vi "SDK Test x64.vi"() -> ()   [LabVIEW 2014]
panel:
  in  "Select Filter Wheel":i32(ring)=1 items=["Filter Wheel 1", "Filter Wheel 2"]
  in  "Select mirror":i32(ring)=1 items=["Mirror 1", "Mirror 2"]
  out "Pixel calibration":dbl
  out "XY Graph":cluster{"Y":dbl[], "Y":dbl[]}[](graph)
  in  "Get calibration":bool
  in  "Pixel Index":i32
  in  "Pixel Width":dbl
  in  "Central WL":dbl
  in  "Pixel Count":i32
  in  "Central Pixel":i32
  out "?":i32
  in  "Grating count":bool
  out "Grating":i32
  in  "Get active grating":bool
  in  "Set active grating":bool
  out "Max WL":dbl
  out "Min WL":dbl
  out "Grooves":i32
  in  "Grating":i32(ring) items=["Grating 1", "Grating 2", "Grating 3", "Grating 4"]
  in  "Reset active grating":bool
  out "Dispersion":dbl format="%.4f"
  out "Error":string
  out "Cur. state":i32(ring) items=["Unknown", "Open", "Close"]
  in  "Set shutter state":bool
  in  "Select shutter state":u32(ring) items=["Open", "Close"]
  out "Cur. filter":i32(ring) items=["Filter1", "Filter2", "Filter3", "Filter4", "Filter5", "Filter6", "Filter7", "Filter8"]
  in  "Set filter":bool
  in  "Select filter state":i32(ring) items=["Filter1", "Filter2", "Filter3", "Filter4", "Filter5", "Filter6", "Filter7", "Filter8"]
  out "Cur. mirror":i32(ring) items=["Undefined"=-1, "Axial port"=0, "Lateral port"=1]
  in  "Set mirror":bool
  in  "Select mirror state":i32(ring)=1 items=["Axial port"=1, "Lateral port"=2]
  in  "Reset":bool
  in  "Set slit width":bool
  out "Slit width":dbl format="%.2f"
  in  "Select slit":i32(ring) items=["Slit 1", "Slit 2", "Slit 3", "Slit 4"]
  in  "New slit width":dbl format="%.2f"
  in  "Stop control":bool
  in  "Set new WL":bool caption="Boolean"
  out "Cur WL":dbl format="%.2f"
  in  "New WL":dbl format="%.2f"
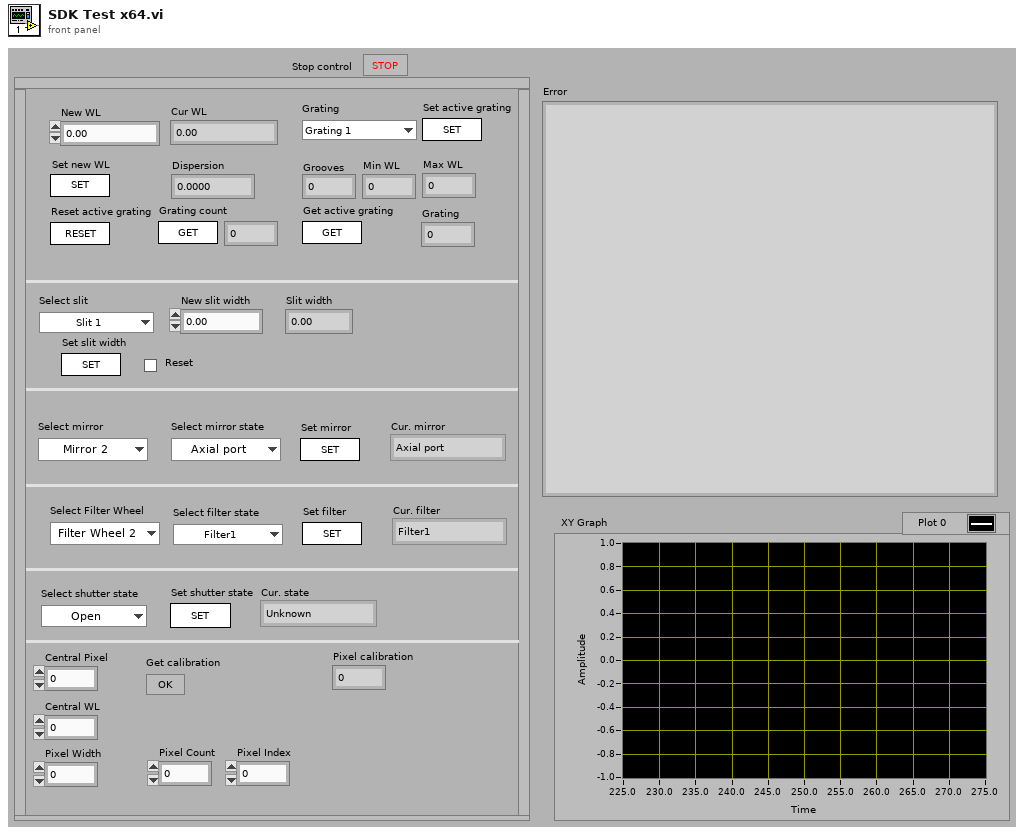
[diagram p1: front panel]
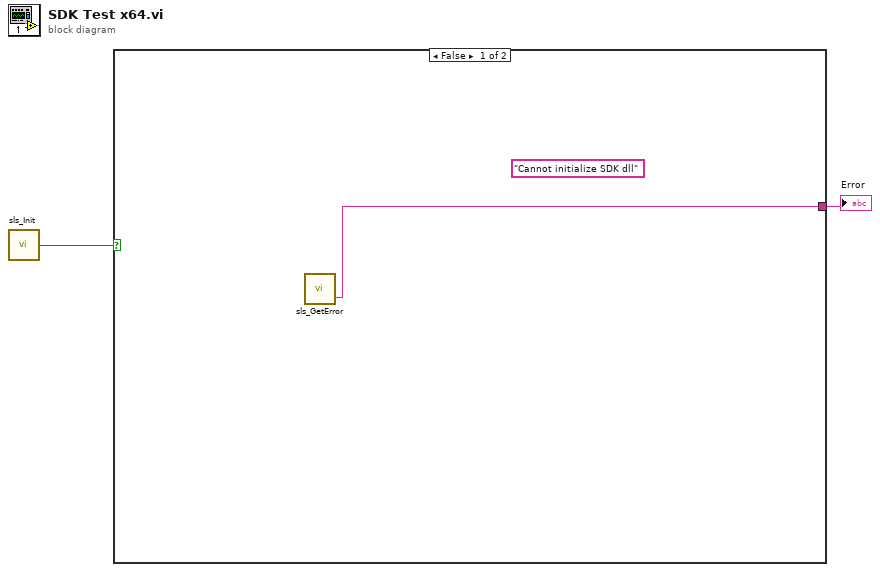
[diagram p0: block diagram]
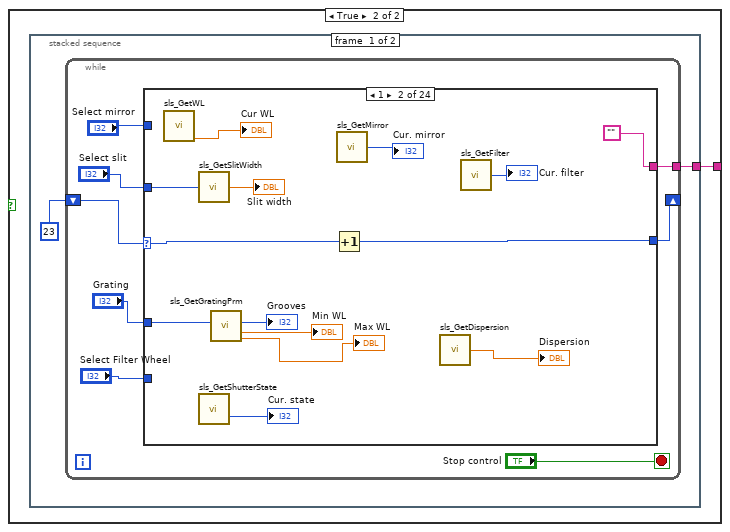
[diagram p2: hidden frame]
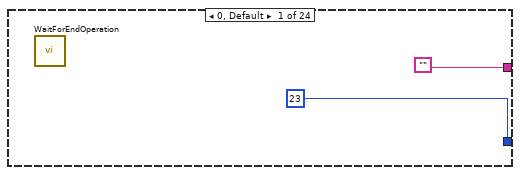
[diagram p3: hidden frame]
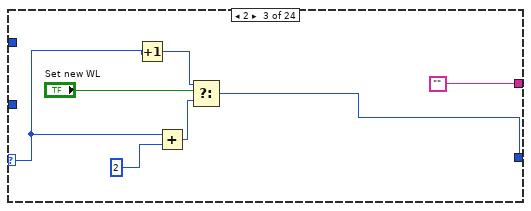
[diagram p4: hidden frame]
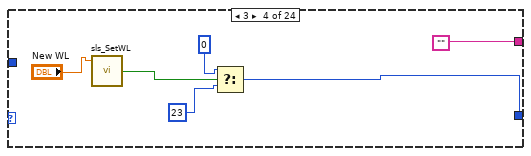
[diagram p5: hidden frame]
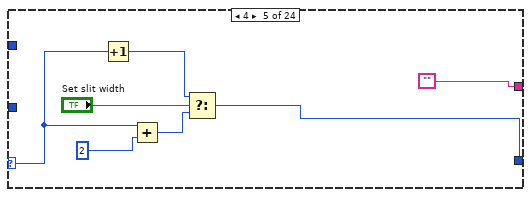
[diagram p6: hidden frame]
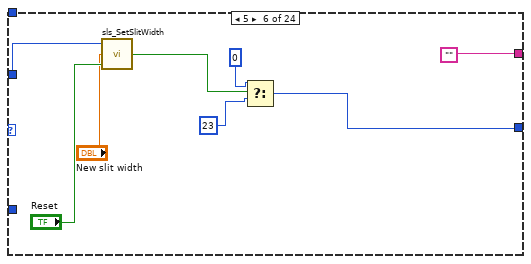
[diagram p7: hidden frame]
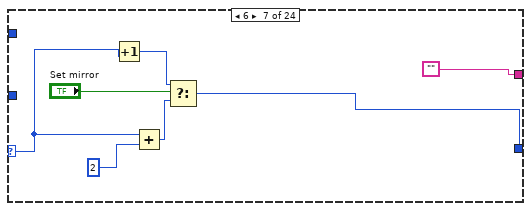
[diagram p8: hidden frame]
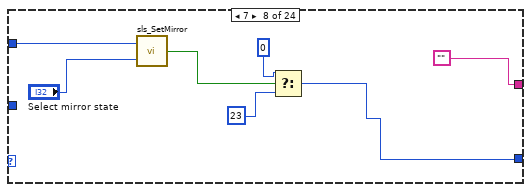
[diagram p9: hidden frame]
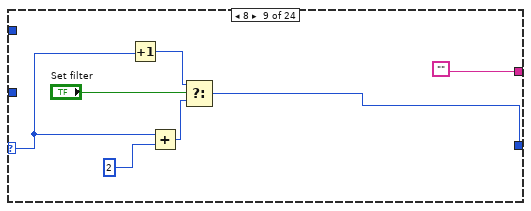
[diagram p10: hidden frame]
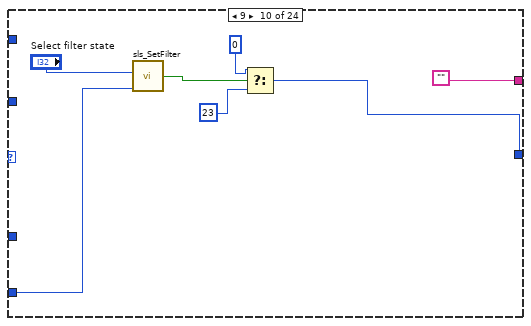
[diagram p11: hidden frame]
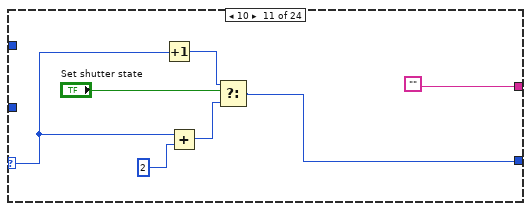
[diagram p12: hidden frame]
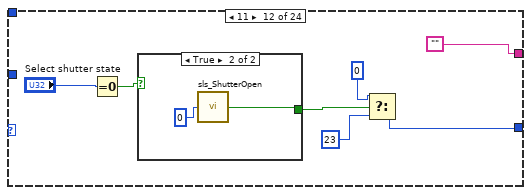
[diagram p13: hidden frame]
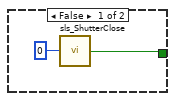
[diagram p14: hidden frame]
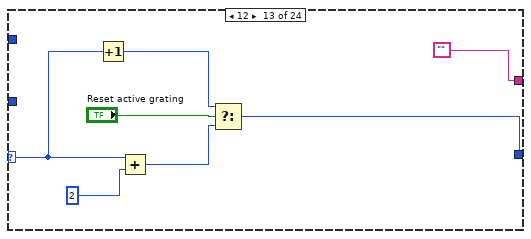
[diagram p15: hidden frame]
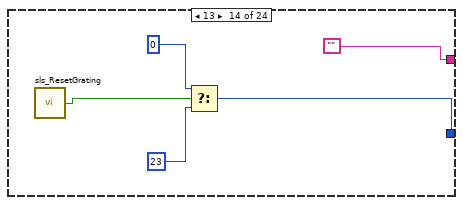
[diagram p16: hidden frame]
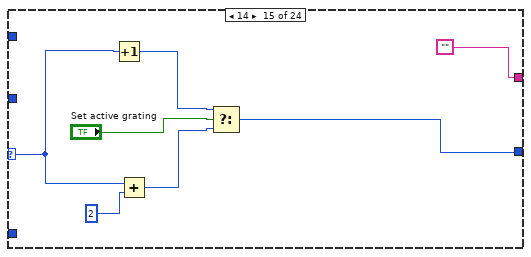
[diagram p17: hidden frame]
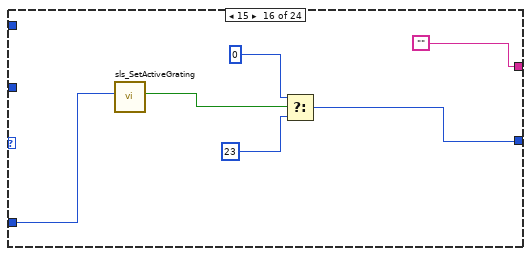
[diagram p18: hidden frame]
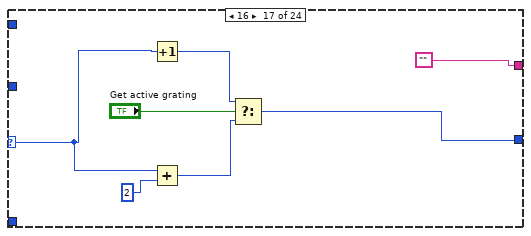
[diagram p19: hidden frame]
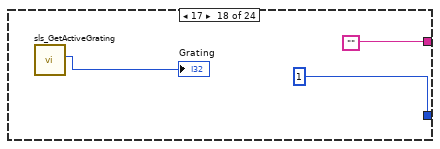
[diagram p20: hidden frame]
diagram:
  n1 = call "sls_Init.vi"() -> ("Result"=w2:bool)  [unwired: 1 in]
  n2 = case shown="False" w2 {
    tunnel: [w3 w4] -> w1
    frame False {
      (unwired) "Cannot initialize SDK dll"
      n3 = call "sls_GetError.vi"() -> ("Error text"=w3:string)  [unwired: 1 in]
    }
    frame True {
      n4 = stacked-sequence {
        tunnel: [w5 _] -> w4
        frame #0 {
          n5 = while {
            shift-right: [w12] -> _
            shift-left: 23 -> [w11]
            tunnel: [w7] -> w5
            stop <- "Stop control" stop-if-true
            n6 = case shown="1" w11 {
              selector: w11 -> [_ w29 w32 _ w45 _ w61 _ w75 _ w91 _ w110 _ w123 _ w135 _ w145 _ w154 _ _ _]
              tunnel: "Select slit" -> [_ w19 _ _ _ w52 _ _ _ _ _ _ _ _ _ _ _ _ _ _ _ _ _ _]
              tunnel: [23 w30 w36 w41 w46 w56 w60 w71 w74 w84 w88 w98 w106 w114 w118 w127 w131 1 w141 1 w151 w166 1 1] -> w12
              tunnel: "Grating" -> [_ w27 _ _ _ _ _ _ _ _ _ _ _ _ _ w125 _ _ _ _ _ _ _ _]
              tunnel: "Select mirror" -> [_ _ _ _ _ _ _ w67 _ _ _ _ _ _ _ _ _ _ _ _ _ _ _ _]
              tunnel: "Select Filter Wheel" -> [_ _ _ _ _ _ _ _ _ w81 _ _ _ _ _ _ _ _ _ _ _ _ _ _]
              tunnel: ["" "" "" "" "" "" "" "" "" "" "" "" "" "" "" "" "" "" "" "" "" "" "" w176] -> w7
              frame 0, Default {
                n7 = call "WaitForEndOperation.vi"() -> ()  [unwired: 1 out]
              }
              frame 1 {
                n8 = call "sls_GetWL.vi"() -> ("Current WL"=→"Cur WL":dbl)  [unwired: 10 in, 1 out]
                n9 = call "sls_GetSlitWidth.vi"("Select slit"=w19) -> ("Slit width"=→"Slit width":dbl)
                n10 = call "sls_GetShutterState.vi"() -> ("Shutter state"=→"Cur. state":i32)
                n11 = call "sls_GetGratingPrm.vi"("Index grating"=w27) -> ("Max WL"=→"Max WL":dbl, "Min WL"=→"Min WL":dbl, "Grooves"=→"Grooves":i32)  [unwired: 7 in, 1 out]
                n12 = Increment(x=w29) -> (x+1=w30:i32)
                n13 = call "sls_GetMirror.vi"() -> ("Mirror position"=→"Cur. mirror":i32)
                n14 = call "sls_GetDispersion.vi"() -> ("Dispersion"=→"Dispersion":dbl)
                n15 = call "sls_GetFilter.vi"() -> ("Filter State"=→"Cur. filter":i32)
              }
              frame 2 {
                n16 = Increment(x=w32) -> (x+1=w35:i32)
                n17 = Add(x=w32, y=2) -> (x+y=w33:i32)
                n18 = Select(t=w35, s="Set new WL", f=w33) -> (s? t:f=w36:i32)
              }
              frame 3 {
                n19 = call "sls_SetWL.vi"("WL"="New WL") -> ("Result"=w40:bool)  [unwired: 2 in]
                n20 = Select(t=0, s=w40, f=23) -> (s? t:f=w41:i32)
              }
              frame 4 {
                n21 = Increment(x=w45) -> (x+1=w49:i32)
                n22 = Add(x=w45, y=2) -> (x+y=w48:i32)
                n23 = Select(t=w49, s="Set slit width", f=w48) -> (s? t:f=w46:i32)
              }
              frame 5 {
                n24 = call "sls_SetSlitWidth.vi"("Reset"="Reset", "Slit width"="New slit width", "Select slit"=w52) -> ("Result"=w55:bool)
                n25 = Select(t=0, s=w55, f=23) -> (s? t:f=w56:i32)
              }
              frame 6 {
                n26 = Increment(x=w61) -> (x+1=w65:i32)
                n27 = Add(x=w61, y=2) -> (x+y=w63:i32)
                n28 = Select(t=w65, s="Set mirror", f=w63) -> (s? t:f=w60:i32)
              }
              frame 7 {
                n29 = call "sls_SetMirror.vi"("Select mirror state"="Select mirror state", "Select Mirror"=w67) -> ("Result"=w69:bool)
                n30 = Select(t=0, s=w69, f=23) -> (s? t:f=w71:i32)
              }
              frame 8 {
                n31 = Increment(x=w75) -> (x+1=w79:i32)
                n32 = Add(x=w75, y=2) -> (x+y=w77:i32)
                n33 = Select(t=w79, s="Set filter", f=w77) -> (s? t:f=w74:i32)
              }
              frame 9 {
                n34 = call "sls_SetFilter.vi"("Select filter state"="Select filter state", "Select filter Wheel"=w81) -> ("Result"=w83:bool)
                n35 = Select(t=0, s=w83, f=23) -> (s? t:f=w84:i32)
              }
              frame 10 {
                n36 = Increment(x=w91) -> (x+1=w93:i32)
                n37 = Add(x=w91, y=2) -> (x+y=w89:i32)
                n38 = Select(t=w93, s="Set shutter state", f=w89) -> (s? t:f=w88:i32)
              }
              frame 11 {
                n39 = Equal To 0?(x="Select shutter state") -> (x = 0?=w96:bool)
                n40 = case shown="True" w96 {
                  tunnel: [w102 w104] -> w95
                  frame False {
                    n41 = call "sls_ShutterClose.vi"("Shutter"=0) -> ("Result"=w102:bool)
                  }
                  frame True {
                    n42 = call "sls_ShutterOpen.vi"("Shutter"=0) -> ("Result"=w104:bool)
                  }
                }
                n43 = Select(t=0, s=w95, f=23) -> (s? t:f=w98:i32)
              }
              frame 12 {
                n44 = Increment(x=w110) -> (x+1=w109:i32)
                n45 = Add(x=w110, y=2) -> (x+y=w108:i32)
                n46 = Select(t=w109, s="Reset active grating", f=w108) -> (s? t:f=w106:i32)
              }
              frame 13 {
                n47 = call "sls_ResetGrating.vi"() -> ("Boolean"=w113:bool)
                n48 = Select(t=0, s=w113, f=23) -> (s? t:f=w114:i32)
              }
              frame 14 {
                n49 = Increment(x=w123) -> (x+1=w121:i32)
                n50 = Add(x=w123, y=2) -> (x+y=w120:i32)
                n51 = Select(t=w121, s="Set active grating", f=w120) -> (s? t:f=w118:i32)
              }
              frame 15 {
                n52 = call "sls_SetActiveGrating.vi"("Grating"=w125) -> ("Boolean"=w126:bool)  [unwired: 10 in]
                n53 = Select(t=0, s=w126, f=23) -> (s? t:f=w127:i32)
              }
              frame 16 {
                n54 = Increment(x=w135) -> (x+1=w134:i32)
                n55 = Add(x=w135, y=2) -> (x+y=w133:i32)
                n56 = Select(t=w134, s="Get active grating", f=w133) -> (s? t:f=w131:i32)
              }
              frame 17 {
                n57 = call "sls_GetActiveGrating.vi"() -> ("Active grating"=→"Grating":i32)  [unwired: 11 in]
              }
              frame 18 {
                n58 = Increment(x=w145) -> (x+1=w143:i32)
                n59 = Add(x=w145, y=2) -> (x+y=w142:i32)
                n60 = Select(t=w143, s="Grating count", f=w142) -> (s? t:f=w141:i32)
              }
              frame 19 {
                n61 = call "sls_GetGratingCount.vi"() -> ("Grating count"=→"?":i32)  [unwired: 11 in]
              }
              frame 20 {
                n62 = Increment(x=w154) -> (x+1=w155:i32)
                n63 = Add(x=w154, y=2) -> (x+y=w153:i32)
                n64 = Select(t=w155, s="Get calibration", f=w153) -> (s? t:f=w151:i32)
              }
              frame 21 {
                n65 = call "sls_GetPxlCalibration.vi"("Central WL"="Central WL", "Pxl Width"="Pixel Width", "Pxl Ind"="Pixel Index", "Central Pxl"="Central Pixel") -> ("Pixel Calibration"=→"Pixel calibration":dbl, "Boolean"=w163:bool)  [unwired: 6 in]
                n66 = call "sls_GetCalibration.vi"("Central Wawelength"="Central WL", "Pixel Pitch"="Pixel Width", "Pixel Count"="Pixel Count", "Central Pixel"="Central Pixel") -> ("Waveform Graph"=w165:dbl[])  [unwired: 5 in, 1 out]
                n67 = Multiply(x=w165, y=0) -> (x*y=w170:dbl[])
                n68 = call "Convert to Dynamic Data"("Array"=w165) -> ("Dynamic Data Type"=w172:dynamicdata)  [unwired: 3 in]
                n69 = call "Convert to Dynamic Data2"("Array"=w170) -> ("Dynamic Data Type"=w169:dynamicdata)  [unwired: 3 in]
                n70 = call "Build XY Graph"("Y Input"=w169, "X Input"=w172) -> ("XY Graph"=→"XY Graph":cluster{"Y":dbl[], "Y":dbl[]}[])  [unwired: 3 in, 6 out]
                n71 = Select(t=0, s=w163, f=23) -> (s? t:f=w166:i32)
              }
              frame 22 {
              }
              frame 23 {
                n72 = call "sls_GetError.vi"() -> ("Error text"=w176:string)  [unwired: 1 in]
              }
            }
          }
        }
        frame #1 {
          n73 = call "WaitForEndOperation.vi"() -> ()  [unwired: 1 out]
        }
      }
    }
  }
  "Error" <- w1
